vi "工單號碼 FGV.vi"(0 "Action":T2=enum."Write", 1 "AddTable 6":string[][](table)=[["工單號碼", "22"], ["產品料號", ""], ["品名", ""], ["作業員", ""], ["生產總數", ""], ["量品數量", ""], ["NG數量", ""], ["良率%", ""], ["", ""], ["", ""], ["", ""], ["", ""], ["", ""], ["", ""], ["", ""], ["", ""], ["", ""], ["", ""], ["", ""], ["", ""], ["", ""], ["", ""], ["", ""], ["", ""], ["", ""], ["", ""], ["", ""]], 3 "工單Data Save Index":T1, 4 "DataIn":string, 5 "工單號碼":string, 6 "Table Load":cluster{"Table Control":string[][]}[](array[cluster]), 7 "error in (no error)":errorcluster) -> (12 "工單號碼的Index":i32, 13 "Read SN Table":string[][](array[string]), 14 "Total Table":cluster{"Table Control":string[][]}[](array[cluster]), 15 "Barcode Array":string[](array[string]), 16 "Read Index Data":string, 17 "Read first table":string[][](array[string]), 18 "工單號碼重複":bool, 19 "error out":errorcluster)   [LabVIEW 2019]
uses:
  Ctrl/MeasureDisplayTab.ctl
  Ctrl/Table Save.ctl
  9377167a-9215-4fe1-b1d7-405c4c1bac97.vi
  09652be0-0e8a-482c-be89-5823cf7997f4.vi
  <vilib>/Utility/xml.llb/Write to XML File(string).vi
  <vilib>/Utility/xml.llb/Read From XML File(string).vi
panel:
  in  "AddTable 2":string[][](table)=[["PCBA BARCODE", ""], ["硬體(Tool初始化)", ""], ["company(Tool初始化)", ""], ["耗電流 uA(電流表)", ""], ["電池負載電壓", ""], ["晶片ID(Tool FORMAT)", ""], ["雷雕ID(TOOl scan、藍芽接收器)", ""], ["Format(Tool FORMAT)", ""], ["Programe(Tool Programe)", ""], ["MAC(藍芽接收器)", ""], ["ID(藍芽接收器)", ""], ["KPA(藍芽接收器)", ""], ["溫度(藍芽接收器)", ""], ["SENSOR電池電壓(藍芽接收器)", ""], ["RSSI(藍芽接收器)", ""], ["SensorType_315(FSK scan)", ""], ["FSKsnVol_315(FSK scan)", ""], ["FSKscanl_315(FSK scan)", ""], ["P_315(Tool FSK scan)", ""], ["T_315(Tool FSK scan)", ""], ["SensorType_433(ASK scan)", ""], ["ASKsnVol_433(ASK scan)", ""], ["ASKscan_433(ASK scan)", ""], ["P_433(ASK scan)", ""], ["T_433(ASK scan)", ""], ["測高Data", ""]]
  in  "Save Index":T3=enum."Format(Tool FORMAT)"
  in  "WriteTable":string[][](table)=[["PCBA BARCODE", ""], ["硬體(Tool初始化)", ""], ["company(Tool初始化)", ""], ["耗電流 uA(電流表)", ""], ["電池負載電壓", ""], ["晶片ID(Tool FORMAT)", ""], ["雷雕ID(TOOl scan、藍芽接收器)", ""], ["Format(Tool FORMAT)", ""], ["Programe(Tool Programe)", ""]]
  out "index of element":i32
  out "LOG":string[][](array[string])
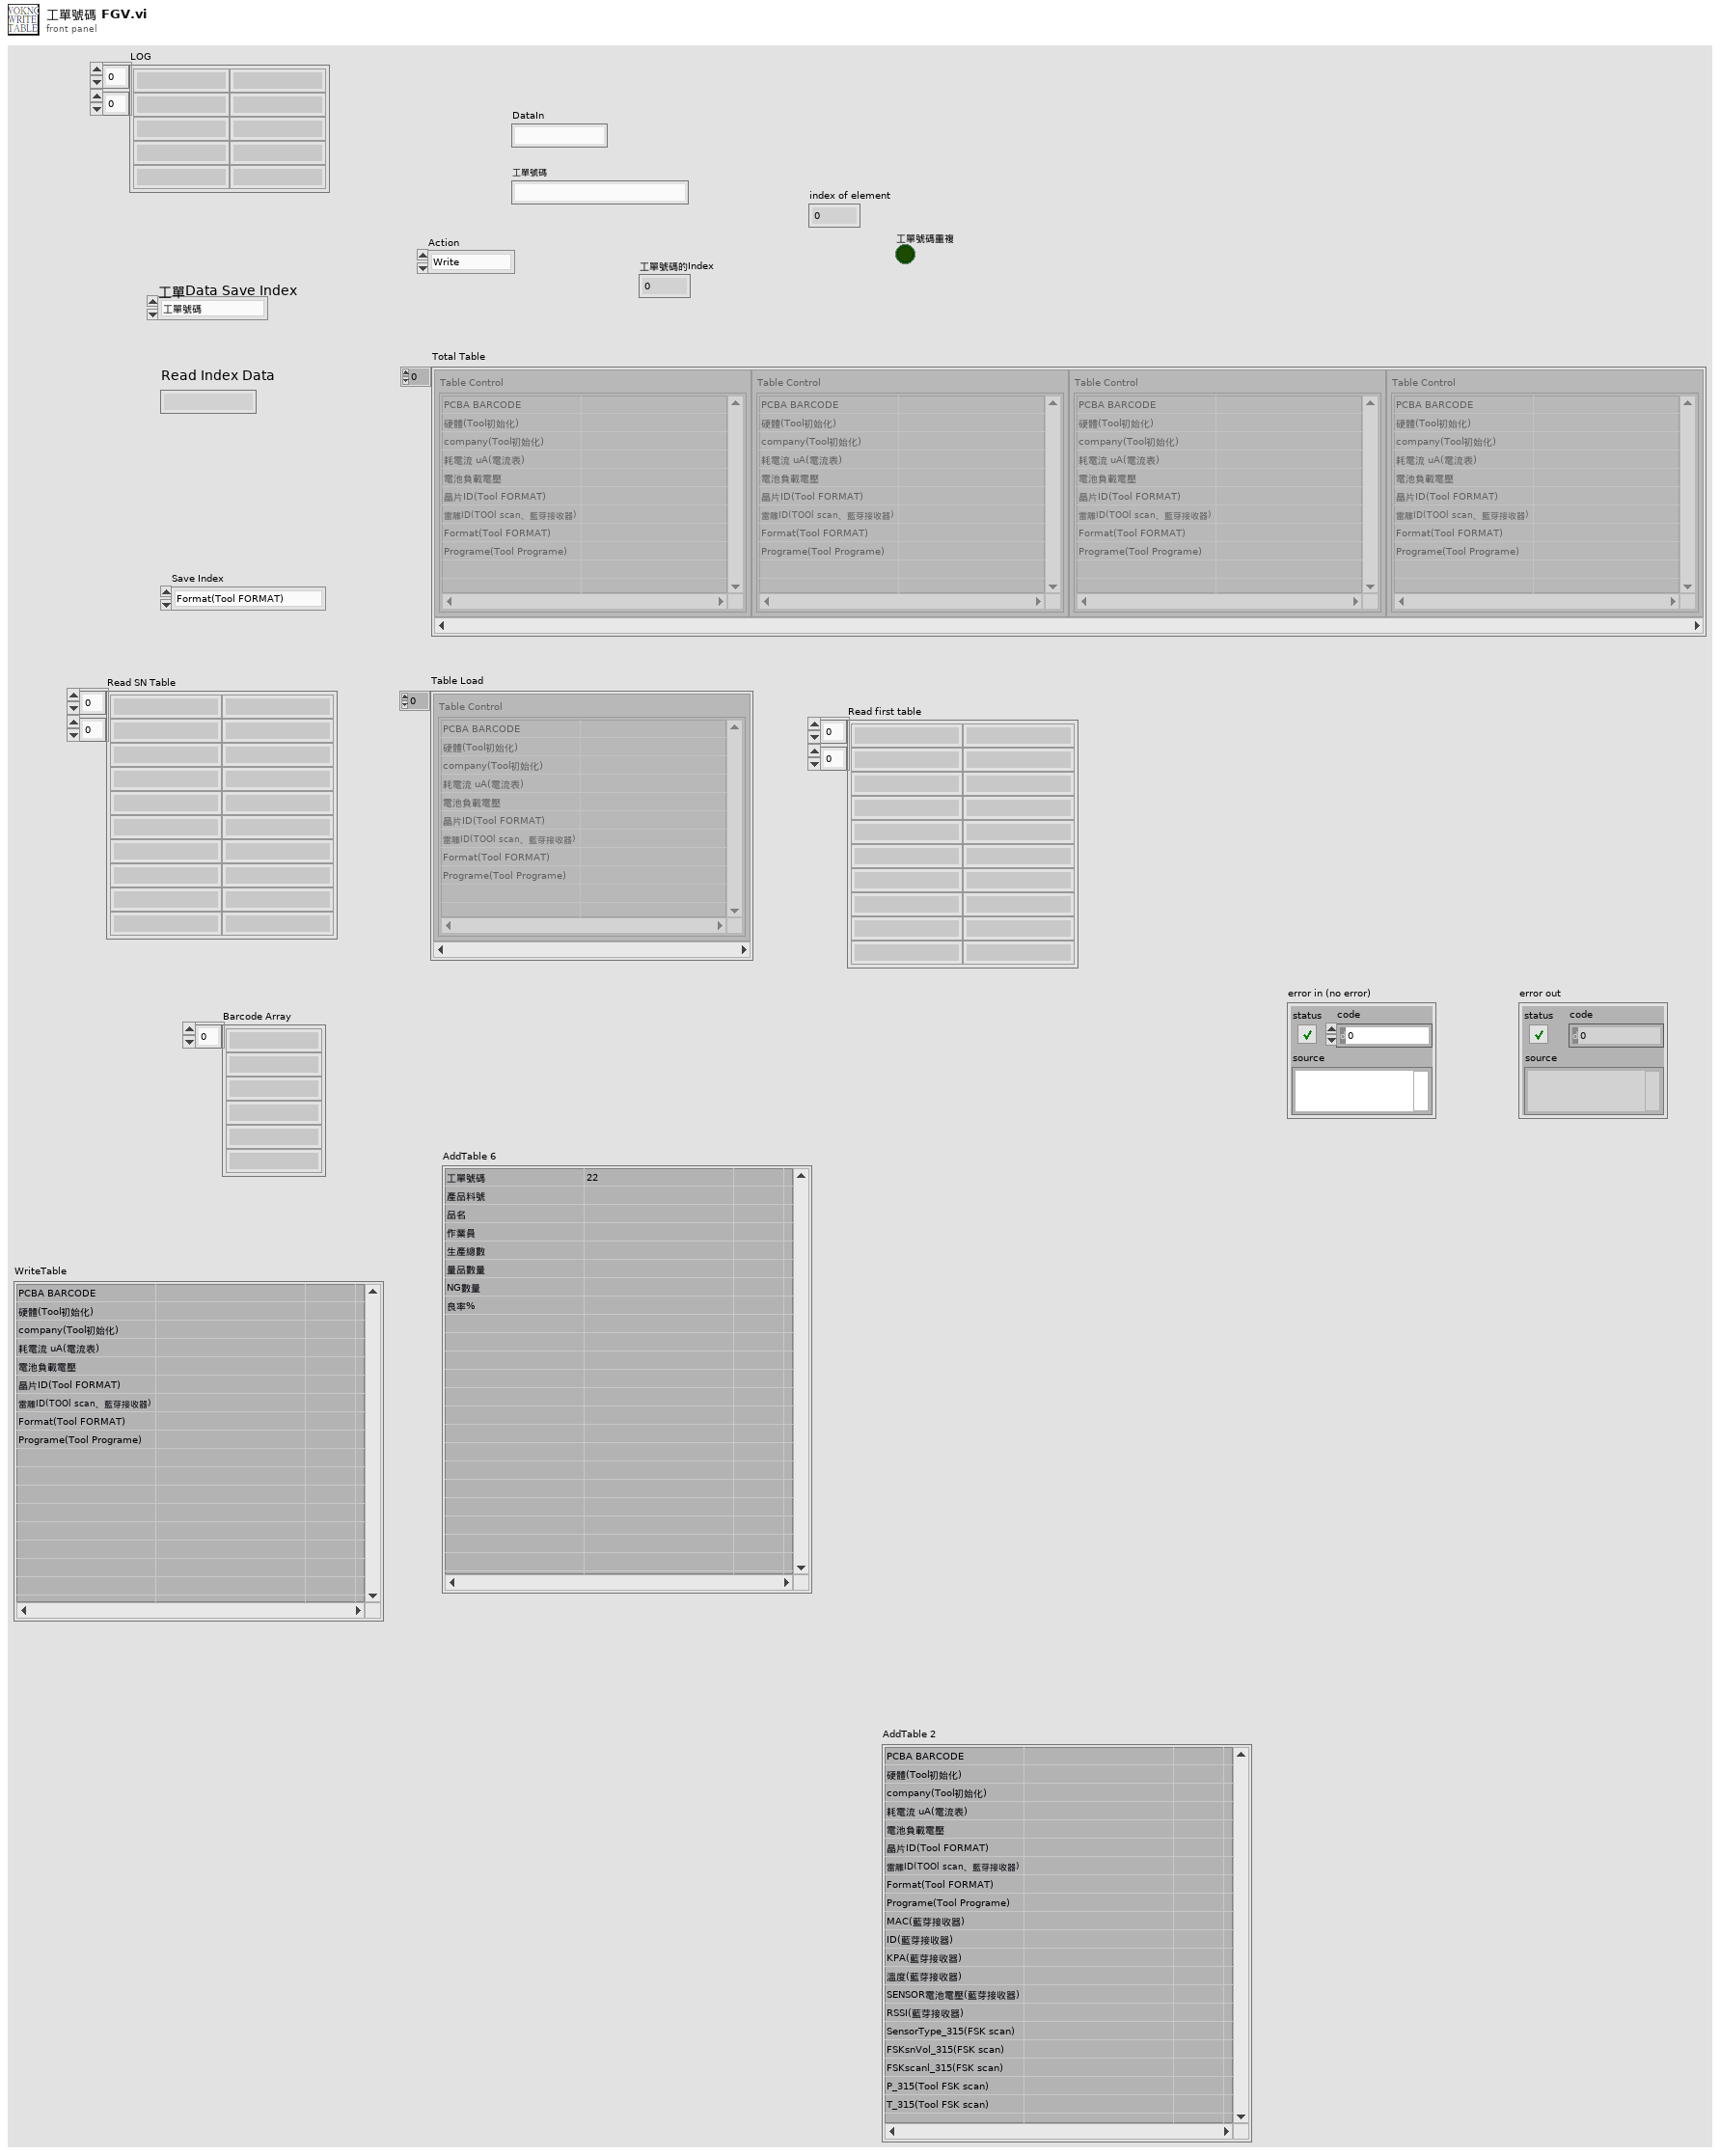
[diagram p1: front panel]
types:
  T1 = typedef "工單號碼_Index.ctl" = enum16{"工單號碼", "產品料號", "品名", "作業員", "生產總數", "量品數量", "NG數量", "良率%"}
  T2 = typedef "Table Save.ctl" = enum16{"initial", "Add", "Write", "Replace", "Delete", "REad", "RedTable", "Load"}
  T3 = typedef "MeasureDisplayTab.ctl" = enum16{"Tray Barcode", "PCBA BARCODE", "硬體(Tool初始化)", "company(Tool初始化)", "耗電流 uA(電流表)", "電池負載電壓", "晶片ID(Tool FORMAT)", "雷雕ID(TOOl scan、藍芽接收器)", "Format(Tool FORMAT)", "Programe(Tool Programe)", "MAC(藍芽接收器)", "ID(藍芽接收器)", "KPA(藍芽接收器)", "溫度(藍芽接收器)", "SENSOR電池電壓(藍芽接收器)", "RSSI(藍芽接收器)", "SensorType_315(FSK scan)", "FSKsnVol_315(FSK scan)", "FSKscanl_315(FSK scan)", "P_315(FSK scan)", "T_315(FSK scan)", "SensorType_433(ASK scan)", "ASKsnVol_433(ASK scan)", "ASKscan_433(ASK scan)", "P_433(ASK scan)", "T_433(ASK scan)", "測高Data"}
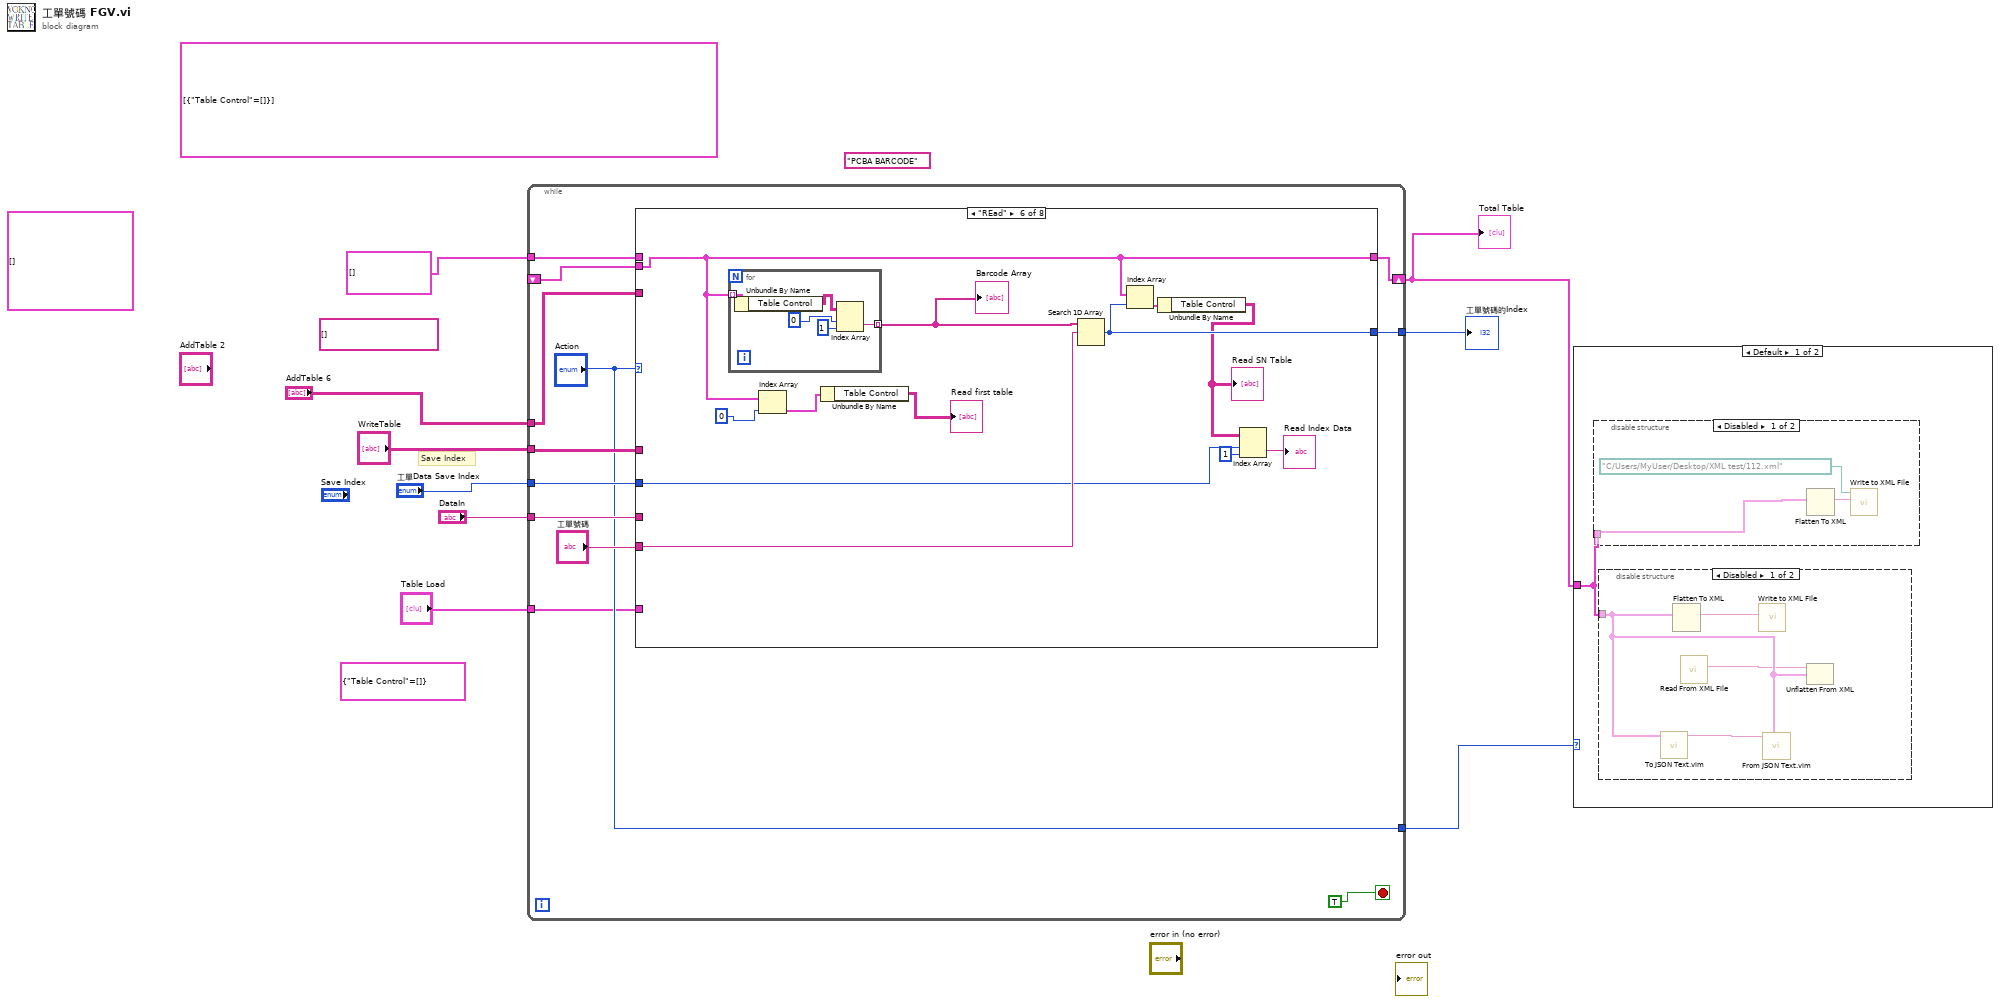
[diagram p0: block diagram]
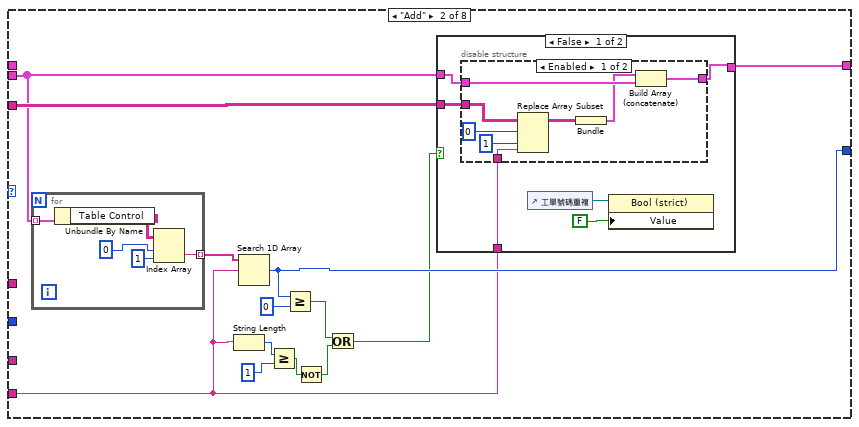
[diagram p6: hidden frame]
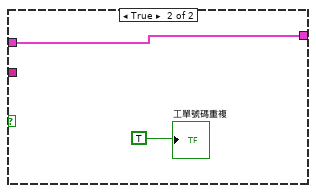
[diagram p8: hidden frame]
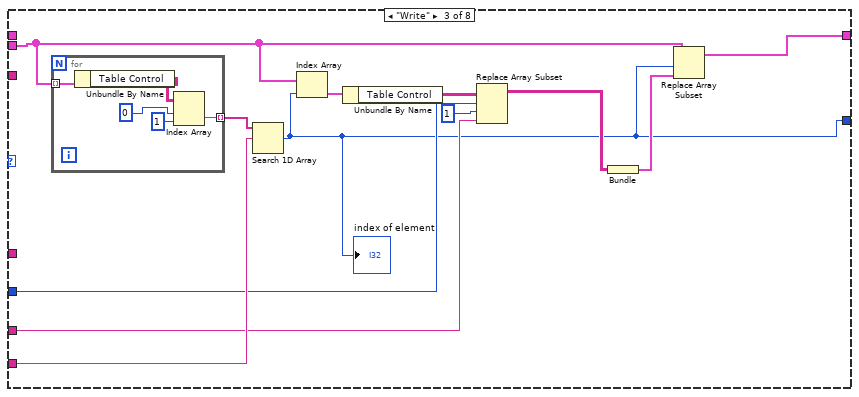
[diagram p9: hidden frame]
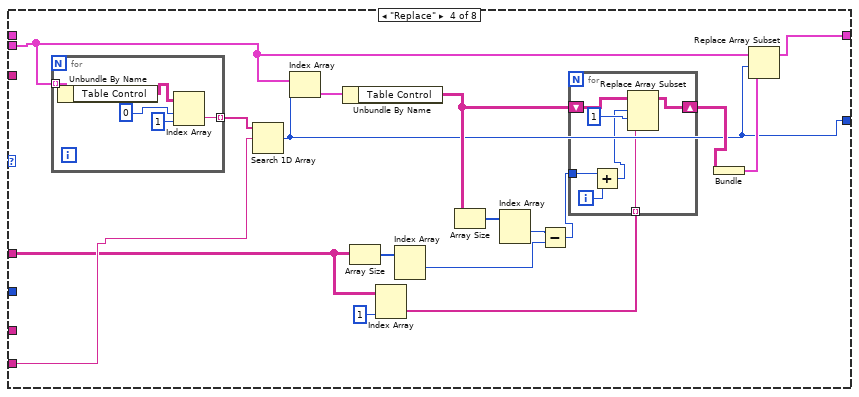
[diagram p10: hidden frame]
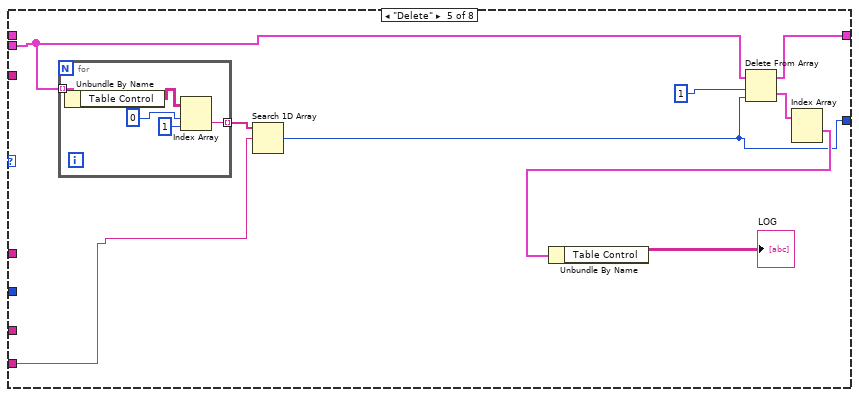
[diagram p11: hidden frame]
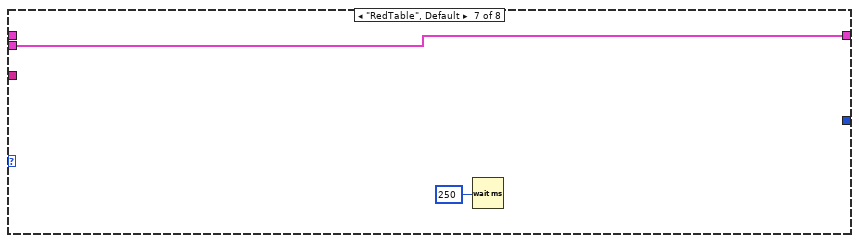
[diagram p12: hidden frame]
diagram:
  (unwired) cluster{"Table Control":string[][]}[] [] ("EnfMeasureTable 2")
  (unwired) cluster{"Table Control":string[][]} {"Table Control"=[]} ("Cluster")
  (unwired) "PCBA BARCODE"
  (unwired) string[][] [] ("Table Control")
  (unwired) cluster{"Table Control":string[][]}[] [{"Table Control"=[]}] ("Array 2")
  # "Save Index"
  n1 = while {
    tunnel: cluster{"Table Control":string[][]}[] [] ("Total Table") -> [w21]
    shift-right: [w20] -> w4
    shift-left: _ -> [w19]
    tunnel: "AddTable 6" -> [w17]
    tunnel: "WriteTable" -> [w14]
    tunnel: ["Action"] -> w8
    tunnel: "工單Data Save Index" -> [w16]
    tunnel: "DataIn" -> [w15]
    tunnel: [w12] -> w6
    tunnel: "Table Load" -> [w10]
    stop <- TRUE stop-if-true
    n2 = case shown="\"REad\"" "Action" {
      tunnel: w21 -> [w22 _ _ _ _ _ _ _]
      tunnel: [w22 w35 w67 w88 w104 w126 w135 w136] -> w20
      tunnel: w17 -> [_ w33 _ _ _ _ _ _]
      tunnel: w19 -> [_ w32 w63 w86 w106 w126 w135 _]
      tunnel: "工單號碼" -> [_ w29 w65 w85 w110 w127 _ _]
      tunnel: w16 -> [_ _ w59 _ _ w119 _ _]
      tunnel: w15 -> [_ _ w58 _ _ _ _ _]
      tunnel: w14 -> [_ _ _ w75 _ _ _ _]
      tunnel: [_ w31 w57 w74 w103 w124 _ _] -> w12
      tunnel: w10 -> [_ _ _ _ _ _ _ w136]
      frame "initial" {
      }
      frame "Add" {
        n3 = for {
          tunnel: w32 -> [w56] mode=indexing
          tunnel: [w52] -> w34 mode=indexing
          n4 = Unbundle By Name(w56) -> ("Table Control"=w55:string[][])
          n5 = Index Array(array=w55, index (row)=0 ("disabled index (col)"), index (col)=1 ("disabled index (col)")) -> (element=w52:string)
        }
        n6 = String Length(string=w29) -> (length=w27:i32)
        n7 = Search 1D Array(1D array=w34, element=w29) -> (index of element=w31:i32)  [unwired: 1 in]
        n8 = Greater Or Equal?(x=w27, y=1) -> (x >= y?=w24:bool)
        n9 = Greater Or Equal?(x=w31, y=0) -> (x >= y?=w28:bool)
        n10 = Not(x=w24) -> (.not. x?=w23:bool)
        n11 = Or(x=w28, y=w23) -> (x .or. y?=w25:bool)
        n12 = case shown="False" w25 {
          tunnel: [w41 w51] -> w35
          tunnel: w33 -> [w40 _]
          tunnel: w29 -> [w39 _]
          tunnel: w32 -> [w36 w51]
          frame False {
            n13 = disable-structure shown="Enabled" {
              disable-tunnel: [w49 _] -> w41
              disable-tunnel: w40 -> [w46 _]
              disable-tunnel: w39 -> [w45 _]
              disable-tunnel: w36 -> [w43 _]
              frame Enabled {
                n14 = Replace Array Subset(array=w46, new element=w45, index (row)=0, index (col)=1) -> (w44:string[][])
                n15 = Bundle("AddTable 6"=w44) -> (w42:cluster{"AddTable 6":string[][]})  [unwired: 1 in]
                n16 = Build Array (concatenate)(w42, w43) -> (w49:cluster{"Table Control":string[][]}[])
              }
              frame Disabled {
              }
            }
            n17 = control-ref of="工單號碼重複"() -> (w38:refnum<vi>)
            n18 = property class="Bool (strict)"(reference=w38, "Value"=FALSE) -> ()  [unwired: 1 in, 2 out]
          }
          frame True {
            "工單號碼重複" <- TRUE
          }
        }
      }
      frame "Write" {
        n19 = for {
          tunnel: w63 -> [w73] mode=indexing
          tunnel: [w69] -> w68 mode=indexing
          n20 = Unbundle By Name(w73) -> ("Table Control"=w72:string[][])
          n21 = Index Array(array=w72, index (row)=0 ("disabled index (col)"), index (col)=1 ("disabled index (col)")) -> (element=w69:string)
        }
        n22 = Search 1D Array(1D array=w68, element=w65) -> (index of element=w57:i32)  [unwired: 1 in]
        "index of element" <- w57
        n23 = Index Array(array=w63, index=w57) -> (element=w64:cluster{"Table Control":string[][]})
        n24 = Unbundle By Name(w64) -> ("Table Control"=w62:string[][])
        n25 = Replace Array Subset(array=w62, new element=w58, index (row)=w59, index (col)=1) -> (w60:string[][])
        n26 = Bundle("Table Control"=w60) -> (w66:cluster{"Table Control":string[][]})  [unwired: 1 in]
        n27 = Replace Array Subset(array=w63, new element=w66, index=w57) -> (w67:cluster{"Table Control":string[][]}[])
      }
      frame "Replace" {
        n28 = for {
          tunnel: w86 -> [w102] mode=indexing
          tunnel: [w98] -> w90 mode=indexing
          n29 = Unbundle By Name(w102) -> ("Table Control"=w101:string[][])
          n30 = Index Array(array=w101, index (row)=0 ("disabled index (col)"), index (col)=1 ("disabled index (col)")) -> (element=w98:string)
        }
        n31 = Search 1D Array(1D array=w90, element=w85) -> (index of element=w74:i32)  [unwired: 1 in]
        n32 = Index Array(array=w86, index=w74) -> (element=w89:cluster{"Table Control":string[][]})
        n33 = Unbundle By Name(w89) -> ("Table Control"=w78:string[][])
        n34 = Array Size(array=w75) -> (size(s)=w82:i32[])
        n35 = Index Array(array=w75, index (col)=1 ("disabled index (col)")) -> (element=w79:string[])  [unwired: 1 in]
        n36 = Index Array(array=w82) -> (element #1=w81:i32)  [unwired: 2 in, 1 out]
        n37 = Array Size(array=w78) -> (size(s)=w83:i32[])
        n38 = Index Array(array=w83) -> (element #1=w77:i32)  [unwired: 2 in, 1 out]
        n39 = Subtract(x=w77, y=w81) -> (x-y=w76:i32)
        n40 = for {
          shift-right: [w97] -> w84
          shift-left: w78 -> [w96]
          tunnel: w76 -> [w93]
          tunnel: w79 -> [w92] mode=indexing
          i -> [w94]
          n41 = Add(x=w93, y=w94) -> (x+y=w91:i32)
          n42 = Replace Array Subset(array=w96, new element=w92, index (row)=w91, index (col)=1 ("disabled index (col)")) -> (w97:string[][])
        }
        n43 = Bundle("Table Control"=w84) -> (w87:cluster{"Table Control":string[][]})  [unwired: 1 in]
        n44 = Replace Array Subset(array=w86, new element=w87, index=w74) -> (w88:cluster{"Table Control":string[][]}[])
      }
      frame "Delete" {
        n45 = for {
          tunnel: w106 -> [w116] mode=indexing
          tunnel: [w112] -> w111 mode=indexing
          n46 = Unbundle By Name(w116) -> ("Table Control"=w115:string[][])
          n47 = Index Array(array=w115, index (row)=0 ("disabled index (col)"), index (col)=1 ("disabled index (col)")) -> (element=w112:string)
        }
        n48 = Search 1D Array(1D array=w111, element=w110) -> (index of element=w103:i32)  [unwired: 1 in]
        n49 = Delete From Array(array=w106, length=1 ("index"), index=w103) -> (deleted portion=w109:cluster{"Table Control":string[][]}[], array with subset deleted=w104:cluster{"Table Control":string[][]}[])
        n50 = Index Array(array=w109) -> (element #1=w108:cluster{"Table Control":string[][]})  [unwired: 2 in, 1 out]
        n51 = Unbundle By Name(w108) -> ("Table Control"=→"LOG":string[][])
      }
      frame "REad" {
        n52 = for {
          tunnel: w126 -> [w133] mode=indexing
          tunnel: [w129] -> w128 mode=indexing
          n53 = Unbundle By Name(w133) -> ("Table Control"=w132:string[][])
          n54 = Index Array(array=w132, index (row)=0 ("disabled index (col)"), index (col)=1 ("disabled index (col)")) -> (element=w129:string)
        }
        "Barcode Array" <- w128
        n55 = Index Array(array=w126, index=0) -> (element=w123:cluster{"Table Control":string[][]})
        n56 = Unbundle By Name(w123) -> ("Table Control"=→"Read first table":string[][])
        n57 = Search 1D Array(1D array=w128, element=w127) -> (index of element=w124:i32)  [unwired: 1 in]
        n58 = Index Array(array=w126, index=w124) -> (element=w125:cluster{"Table Control":string[][]})
        n59 = Unbundle By Name(w125) -> ("Table Control"=w120:string[][])
        "Read SN Table" <- w120
        n60 = Index Array(array=w120, index (row)=w119, index (col)=1 ("disabled index (col)")) -> (element=→"Read Index Data":string)
      }
      frame "RedTable", Default {
        n61 = Wait (ms)(milliseconds to wait=250) -> ()  [unwired: 1 out]
      }
      frame "Load" {
      }
    }
  }
  "工單號碼的Index" <- w6
  "Total Table" <- w4
  n62 = case shown="Default" w8 {
    tunnel: w4 -> [w137 _]
    frame Default {
      n63 = disable-structure shown="Disabled" {
        disable-tunnel: w137 -> [w138 _]
        frame Disabled {
          n64 = Flatten To XML(anything=w138) -> (xml string=w140:string)
          n65 = call-poly <vilib>:"Write to XML File.vi"("XML Input"=w140, "XML File Path"=path "C:/Users/MyUser/Desktop/XML test/112.xml") -> ()  [unwired: 7 in, 3 out]
        }
        frame Enabled {
        }
      }
      n66 = disable-structure shown="Disabled" {
        disable-tunnel: w137 -> [w143 _]
        frame Disabled {
          n67 = call "To JSON Text.vim"("Anything"=w143) -> ("<JSON>"=w144:string)  [unwired: 9 in, 1 out]
          n68 = Flatten To XML(anything=w143) -> (xml string=w141:string)
          n69 = call-poly <vilib>:"Read From XML File.vi"() -> ("XML Elements"=w142:string)  [unwired: 9 in, 2 out]
          n70 = call-poly <vilib>:"Write to XML File.vi"("XML Input"=w141) -> ()  [unwired: 8 in, 3 out]
          n71 = call "From JSON Text.vim"("Data Type and Default Value"=w143, "JSON"=w144) -> ()  [unwired: 8 in, 2 out]
          n72 = Unflatten From XML(xml string=w142, type=w143) -> ()  [unwired: 1 in, 2 out]
        }
        frame Enabled {
        }
      }
    }
    frame "initial", "REad" {
    }
  }
